vi "Sentran Accuracy Test SAA.vi"(8 "error in (no error)":errorcluster, 10 "Model in":refnum<class "Model.lvclass">, 11 "Test Actuator State in":refnum<class "Test Actuator State.lvclass">) -> (0 "error out":errorcluster, 1 "Pass":bool, 2 "Model out":refnum<class "Model.lvclass">, 3 "Test Actuator State out":refnum<class "Test Actuator State.lvclass">)   [LabVIEW 2016]
uses:
  Model/Model/Model.lvclass
  Typedefs/ActuatorSetPoints.ctl
  <vilib>/platform/TimedLoop/XDataNode/XDataNode.xnode
  <vilib>/Platform/TimedLoop/XDataNode/nitl_modes.ctl
  <vilib>/Platform/TimedLoop/XDataNode/XDNodeRunTimeDep.lvlib
  <vilib>/Platform/TimedLoop/XDataNode/wakeup.ctl
  <vilib>/Platform/TimedLoop/XDataNode/timing_clust.ctl
  Test Actuator State.lvclass
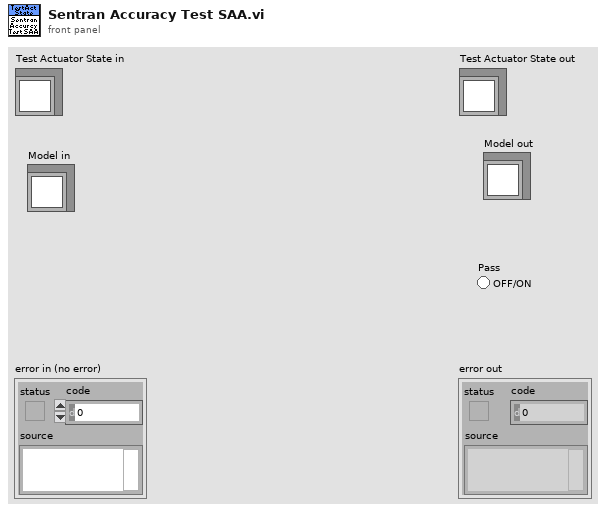
[diagram p1: front panel]
types:
  T1 = typedef "SentranAccuracyTestSettings.ctl" = cluster{"Force Tolerance (N)":dbl, "Force Modifies (%)":dbl[], "Process Time (s)":dbl, "Sample Time (s)":dbl, "Max Moment (NM)":dbl}
  T2 = typedef "ForcePair.ctl" = cluster{"Axial Force":dbl, "Lateral Force":dbl}
  T3 = typedef "ActuatorSetPoints.ctl" = cluster{"Axial Force":dbl, "Lateral Force":dbl, "FC1 Force":dbl, "FC2 Force":dbl}
  T4 = typedef "XDNodeRunTimeDep.lvlib/timing_clust.ctl" = cluster{"Expected End [f-1]":u64, "Actual End [f-1]":u64, "Finished Late? [f-1]":bool, "Expected End [i-1]":u64, "Actual End [i-1]":u64, "Finished Late? [i-1]":bool, "Expected Start [i]":u64, "Actual Start [i]":u64, "Expected Start [f]":u64, "Actual Start [f]":u64, "Source Name":string, "Structure Name":string, "Period":i64, "Deadline":i64, "Offset":i64, "Start":i64, "Priority":i32, "Timeout":i32, "Mode":T5, "Wakeup Reason":T6, "Error":errorcluster, "Source Type":string, "Secondary Source Type":string, "Global End Time":u64, "Global Start Time":u64, "Frame Duration":u64, "Iteration Duration":u64, "Assigned CPU":i32, "I/O Scan Engine Mode":u32}
  T5 = typedef "XDNodeRunTimeDep.lvlib/nitl_modes.ctl" = enum32{"No Change", "Process missed periods, maintain original phase", "Discard missed periods, maintain original phase", "Process missed periods, ignore original phase", "Discard missed periods, ignore original phase"}
  T6 = typedef "XDNodeRunTimeDep.lvlib/wakeup.ctl" = enum32{"Normal", "Aborted", "Asynchronous wakeup", "Timing source error", "Timed loop error", "Timeout"}
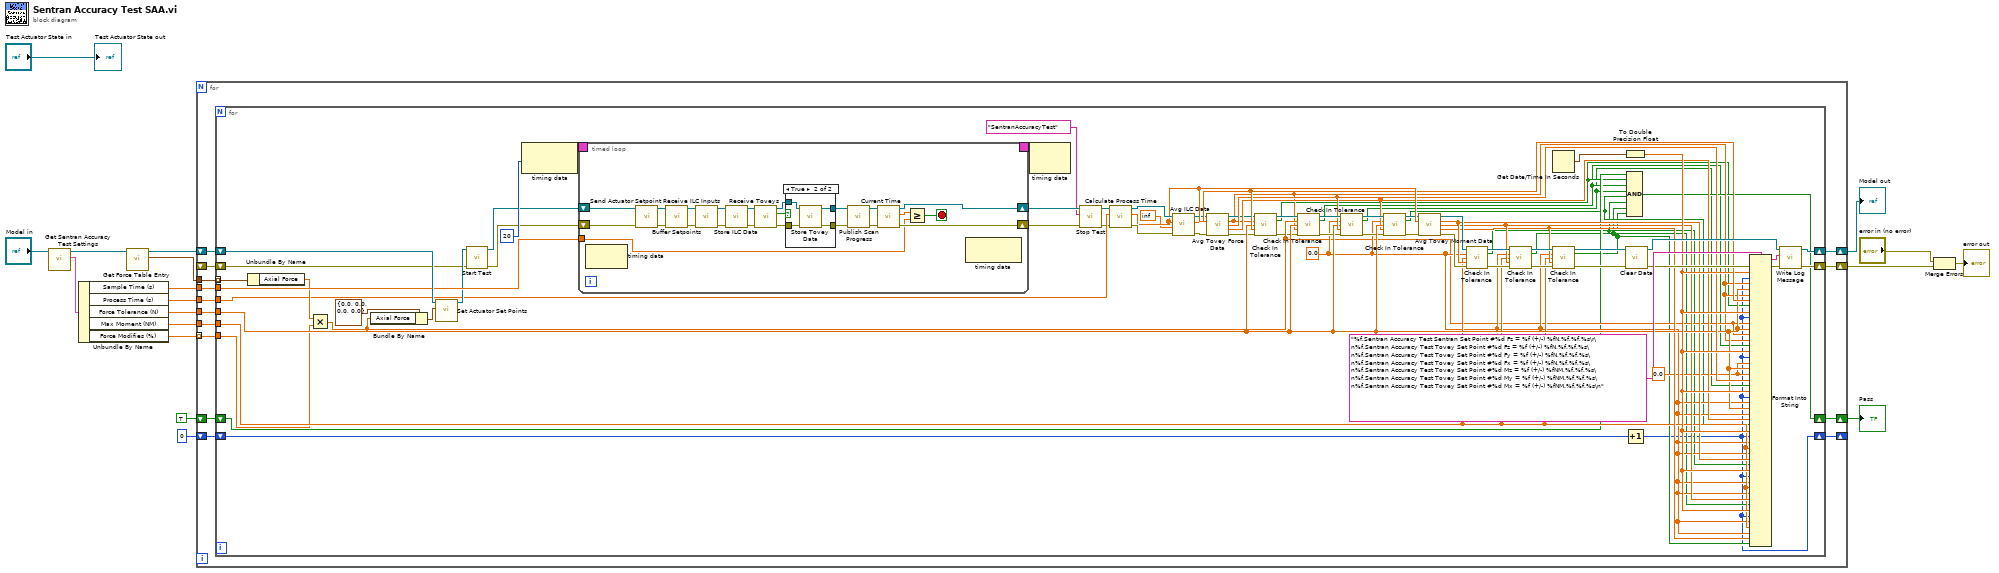
[diagram p0: block diagram]
diagram:
  n1 = call "Get Sentran Accuracy Test Settings.vi"("Model in"="Model in") -> ("Sentran Accuracy Test Settings"=w12:T1, "Model out"=w4:refnum<class "Model.lvclass">)  [unwired: 9 in]
  n2 = Unbundle By Name(w12) -> ("Sample Time (s)"=w11:dbl, "Process Time (s)"=w10:dbl, "Force Tolerance (N)"=w9:dbl, "Max Moment (NM)"=w8:dbl, "Force Modifies (%)"=w7:dbl[])
  n3 = call "Get Force Table Entry.vi"("Model in"=w4) -> ("Entry"=w3:T2[], "Model out"=w2:refnum<class "Model.lvclass">)  [unwired: 8 in, 1 out]
  n4 = for {
    tunnel: w11 -> [w29]
    tunnel: w10 -> [w28]
    tunnel: w9 -> [w27]
    tunnel: w8 -> [w26]
    shift-right: [w31] -> w15
    shift-left: w2 -> [w32]
    shift-right: [w30] -> w14
    shift-left: _ -> [w25]
    tunnel: w7 -> [w24] mode=indexing
    shift-right: [w22] -> w5
    shift-left: TRUE -> [w23]
    tunnel: w3 -> [w21]
    shift-right: [w19] -> _
    shift-left: 0 -> [w20]
    n5 = for {
      shift-right: [w104] -> w31
      shift-left: w32 -> [w107]
      tunnel: w29 -> [w106]
      tunnel: w28 -> [w51]
      tunnel: w27 -> [w88]
      shift-right: [w97] -> w30
      shift-left: w25 -> [w54]
      tunnel: w26 -> [w71]
      tunnel: w24 -> [w56]
      shift-right: [w44] -> w22
      shift-left: w23 -> [w43]
      tunnel: w21 -> [w35] mode=indexing
      shift-right: [w33] -> w19
      shift-left: w20 -> [w34]
      w45 = 0.0 ("input 17")
      w70 = 0.0
      n6 = Unbundle By Name(w35) -> ("Axial Force"=w68:dbl)
      n7 = Multiply(x=w68, y=w56) -> (x*y=w67:dbl)
      n8 = Bundle By Name(cluster=T3 {"Axial Force"=0.0, "Lateral Force"=0.0, "FC1 Force"=0.0, "FC2 Force"=0.0} ("Actuator Set Points"), "Axial Force"=w67) -> (w101:T3)
      n9 = call "Set Actuator Set Points.vi"("Actuator Set Points"=w101, "Model in"=w107) -> ("Model out"=w55:refnum<class "Model.lvclass">)  [unwired: 9 in]
      n10 = call "Start Test.vi"("error in (no error)"=w54, "Model in"=w55) -> ("error out"=w53:errorcluster, "Model out"=w52:refnum<class "Model.lvclass">)  [unwired: 8 in]
      n11 = node-c288(i64 20 ("Period")) -> (w59:T4)
      n12 = timed-loop {
        shift-right: [w126] -> w50
        shift-left: w52 -> [w130]
        shift-right: [w125] -> w48
        shift-left: w53 -> [w128]
        tunnel: w106 -> [w123]
        timing: w59 -> [_]
        timing-out: [_] -> w58
        stop <- w122 stop-if-true
        n13 = node-c288() -> ()  [unwired: 1 in, 1 out]
        n14 = call "Send Actuator Setpoint.vi"("error in (no error)"=w128, "Model in"=w130) -> ("error out"=w110:errorcluster, "Model out"=w112:refnum<class "Model.lvclass">)  [unwired: 8 in]
        n15 = call "Buffer Setpoints.vi"("error in (no error)"=w110, "Model in"=w112) -> ("error out"=w109:errorcluster, "Model out"=w111:refnum<class "Model.lvclass">)  [unwired: 8 in]
        n16 = call "Receive ILC Inputs.vi"("error in (no error)"=w109, "Model in"=w111) -> ("error out"=w127:errorcluster, "Model out"=w129:refnum<class "Model.lvclass">)  [unwired: 8 in]
        n17 = call "Store ILC Data.vi"("error in (no error)"=w127, "Model in"=w129) -> ("error out"=w120:errorcluster, "Model out"=w121:refnum<class "Model.lvclass">)  [unwired: 8 in]
        n18 = call "Receive Toveys.vi"("error in (no error)"=w120, "Model in"=w121) -> ("error out"=w118:errorcluster, "Data Received"=w117:bool, "Model out"=w119:refnum<class "Model.lvclass">)  [unwired: 7 in]
        n19 = case shown="True" w117 {
          tunnel: w119 -> [w134 w138]
          tunnel: w118 -> [w133 w137]
          tunnel: [w133 w136] -> w113
          tunnel: [w134 w135] -> w116
          frame False {
          }
          frame True {
            n20 = call "Store Tovey Data.vi"("error in (no error)"=w137, "Model in"=w138) -> ("error out"=w136:errorcluster, "Model out"=w135:refnum<class "Model.lvclass">)  [unwired: 8 in]
          }
        }
        n21 = call "Publish Scan Progress.vi"("error in (no error)"=w113, "Model in"=w116) -> ("error out"=w114:errorcluster, "Model out"=w115:refnum<class "Model.lvclass">)  [unwired: 8 in]
        n22 = call "Current Time.vi"("error in (no error)"=w114, "Model in"=w115) -> ("error out"=w125:errorcluster, "Time"=w124:dbl, "Model out"=w126:refnum<class "Model.lvclass">)  [unwired: 7 in]
        n23 = Greater Or Equal?(x=w124, y=w123) -> (x >= y?=w122:bool)
        n24 = node-c288() -> ()  [unwired: 1 in, 1 out]
      }
      n25 = node-c288(w58) -> ()  [unwired: 1 out]
      n26 = call "Stop Test.vi"("error in (no error)"=w48, "Test"="SentranAccuracyTest", "Model in"=w50) -> ("error out"=w47:errorcluster, "Model out"=w49:refnum<class "Model.lvclass">)  [unwired: 7 in]
      n27 = call "Calculate Process Time.vi"("error in (no error)"=w47, "Seconds"=w51, "Model in"=w49) -> ("error out"=w95:errorcluster, "Time"=w94:dbl, "Model out"=w96:refnum<class "Model.lvclass">)  [unwired: 6 in]
      n28 = call "Avg ILC Data.vi"("error in (no error)"=w95, "Before This Time"=inf, "After This Time"=w94, "Model in"=w96) -> ("error out"=w63:errorcluster, "Force"=w93:dbl, "Model out"=w66:refnum<class "Model.lvclass">)  [unwired: 5 in]
      n29 = call "Avg Tovey Force Data.vi"("Model in"=w66, "After This Time"=w94, "error in (no error)"=w63) -> ("Model out"=w65:refnum<class "Model.lvclass">, "Fz"=w60:dbl, "Fy"=w90:dbl, "Fx"=w81:dbl, "error out"=w62:errorcluster)  [unwired: 8 in]
      n30 = call "Check In Tolerance.vi"("Model in"=w65, "Expected"=w60, "Tolerance"=w88, "Actual"=w93, "error in (no error)"=w62) -> ("Model out"=w64:refnum<class "Model.lvclass">, "Pass"=w42:bool, "error out"=w61:errorcluster)  [unwired: 8 in]
      n31 = call "Check In Tolerance.vi"("Model in"=w64, "Expected"=w67, "Tolerance"=w88, "Actual"=w60, "error in (no error)"=w61) -> ("Model out"=w91:refnum<class "Model.lvclass">, "Pass"=w41:bool, "error out"=w87:errorcluster)  [unwired: 8 in]
      n32 = call "Check In Tolerance.vi"("Model in"=w91, "Expected"=w70, "Tolerance"=w88, "Actual"=w90, "error in (no error)"=w87) -> ("Model out"=w89:refnum<class "Model.lvclass">, "Pass"=w40:bool, "error out"=w86:errorcluster)  [unwired: 8 in]
      n33 = call "Check In Tolerance.vi"("Model in"=w89, "Expected"=w70, "Tolerance"=w88, "Actual"=w81, "error in (no error)"=w86) -> ("Model out"=w84:refnum<class "Model.lvclass">, "Pass"=w39:bool, "error out"=w85:errorcluster)  [unwired: 8 in]
      n34 = call "Avg Tovey Moment Data.vi"("Model in"=w84, "After This Time"=w94, "error in (no error)"=w85) -> ("Model out"=w83:refnum<class "Model.lvclass">, "Mz"=w80:dbl, "My"=w77:dbl, "Mx"=w76:dbl, "error out"=w82:errorcluster)  [unwired: 8 in]
      n35 = call "Check In Tolerance.vi"("Model in"=w83, "Expected"=w70, "Tolerance"=w71, "Actual"=w80, "error in (no error)"=w82) -> ("Model out"=w79:refnum<class "Model.lvclass">, "Pass"=w38:bool, "error out"=w74:errorcluster)  [unwired: 8 in]
      n36 = call "Check In Tolerance.vi"("Model in"=w79, "Expected"=w70, "Tolerance"=w71, "Actual"=w77, "error in (no error)"=w74) -> ("Model out"=w78:refnum<class "Model.lvclass">, "Pass"=w37:bool, "error out"=w73:errorcluster)  [unwired: 8 in]
      n37 = Get Date/Time In Seconds() -> (seconds since 1Jan1904=w102:timestamp)
      n38 = call "Check In Tolerance.vi"("Model in"=w78, "Expected"=w70, "Tolerance"=w71, "Actual"=w76, "error in (no error)"=w73) -> ("Model out"=w75:refnum<class "Model.lvclass">, "Pass"=w36:bool, "error out"=w72:errorcluster)  [unwired: 8 in]
      n39 = To Double Precision Float(number=w102) -> (double precision float=w92:dbl)
      n40 = Increment(x=w34) -> (x+1=w33:i32)
      n41 = call "Clear Data.vi"("error in (no error)"=w72, "Model in"=w75) -> ("error out"=w99:errorcluster, "Model out"=w105:refnum<class "Model.lvclass">)  [unwired: 8 in]
      n42 = Compound Arithmetic op=AND(w43, w42, w41, w40, w39, w38, w37, w36) -> (w44:bool)
      n43 = Format Into String(format string="%f,Sentran Accuracy Test Sentran Set Point #%d Fz = %f (+/-) %fN,%f,%f,%s\r\n%f,Sentran Accuracy Test Tovey Set Point #%d Fz = %f (+/-) %fN,%f,%f,%s\n%f,Sentran Accuracy Test Tovey Set Point #%d Fy = %f (+/-) %fN,%f,%f,%s\n%f,Sentran Accuracy Test Tovey Set Point #%d Fx = %f (+/-) %fN,%f,%f,%s\n%f,Sentran Accuracy Test Tovey Set Point #%d Mz = %f (+/-) %fNM,%f,%f,%s\n%f,Sentran Accuracy Test Tovey Set Point #%d My = %f (+/-) %fNM,%f,%f,%s\n%f,Sentran Accuracy Test Tovey Set Point #%d Mx = %f (+/-) %fNM,%f,%f,%s\n", error in=w99, w92, w33, w60, w88, w60, w93, w42, w92, w33, w67, w88, w67, w60, w41, w92, w33, w45, w88, w45, w90, w40, w92, w33, w70, w88, w70, w81, w39, w92, w33, w70, w71, w70, w80, w38, w92, w33, w70, w71, w70, w77, w37, w92, w33, w70, w71, w70, w76, w36) -> (resulting string=w100:string, error out=w98:errorcluster)  [unwired: 1 in]
      n44 = call "Write Log Message.vi"("error in (no error)"=w98, "Message"=w100, "Model in"=w105) -> ("error out"=w97:errorcluster, "Model out"=w104:refnum<class "Model.lvclass">)  [unwired: 7 in]
    }
  }
  "Model out" <- w15
  "Pass" <- w5
  n45 = Merge Errors("error in (no error)", w14) -> (→"error out":errorcluster)
  "Test Actuator State out" <- "Test Actuator State in"
